vi "PushGoldenSingleData.vi"(8 "errin":errorcluster, 9 "Value":string, 10 "TestNum":string, 11 "SN":string) -> (0 "errout":errorcluster, 3 "String out":string)   [LabVIEW 2020]
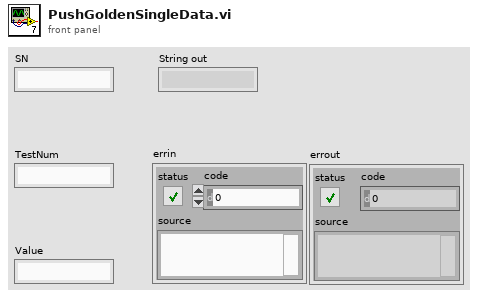
[diagram p1: front panel]
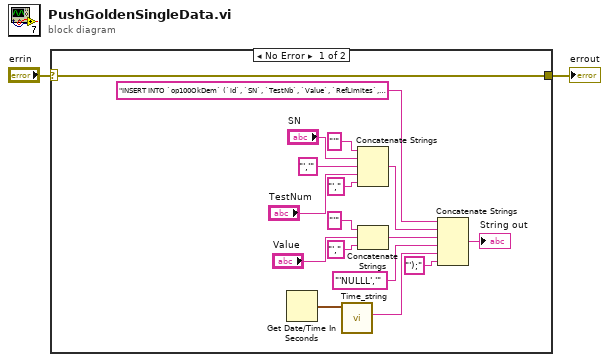
[diagram p0: block diagram]
diagram:
  n1 = case shown="No Error" "errin" {
    selector: "errin" -> [w3 w20]
    tunnel: [w3 w20] -> w1
    frame No Error {
      n2 = Get Date/Time In Seconds() -> (seconds since 1Jan1904=w8:timestamp)
      n3 = call <userlib>:"Time_string.vi"("h in"=w8) -> ("heure sql"=w11:string)  [unwired: 9 in, 1 out]
      n4 = Concatenate Strings("'" ("string"), "SN", "','" ("string"), "TestNum", "'," ("string")) -> (w6:string)
      n5 = Concatenate Strings("'" ("chaîne"), "Value", "'," ("string")) -> (w9:string)
      n6 = Concatenate Strings("INSERT INTO `op100OkDem` (`id`, `SN`, `TestNb`, `Value`, `RefLimites`, `Date`) VALUES (NULL, " ("chaîne"), w6, w9, "'NULLL','" ("string"), w11, "');" ("string")) -> (→"String out":string)
    }
    frame Error {
    }
  }
  "errout" <- w1
